vi "Eval X-Y-Z(a,t1,t2) Prep.vi"(0 "End":dbl[](array[numeric])=[1.0, 1.0] format="%.2f", 5 "Formulas":string[](array[string])=["", "", ""], 7 "Variables":string[](array[string])=["t1", "t2"], 9 "Parameters":cluster{string, dbl}[](array[cluster]) {"?" format="%.2f"}, 11 "Start":dbl[](array[numeric])=[0.0, 0.0] format="%.2f") -> (4 "Formulas":string[](array[string]), 6 "End":dbl[](array[numeric]) format="%.2f", 8 "time [msec]":u32, 10 "error (general)":bool, 12 "Variables":string[](array[string]), 13 "Start":dbl[](array[numeric]) format="%.2f", 14 "Parameters":cluster{string, dbl}[](array[cluster]) {"?" format="%.2f"}, 15 "specific error situation":bool)   [LabVIEW 2017, in "NI_Gmath.lvlib"]
uses:
  NI_Gmath.lvlib
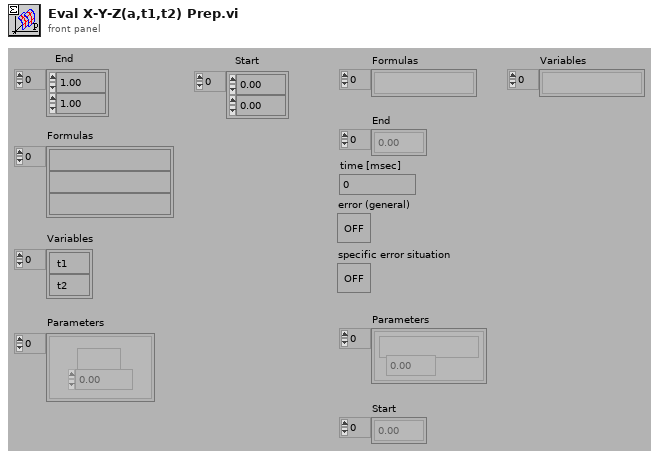
[diagram p1: front panel]
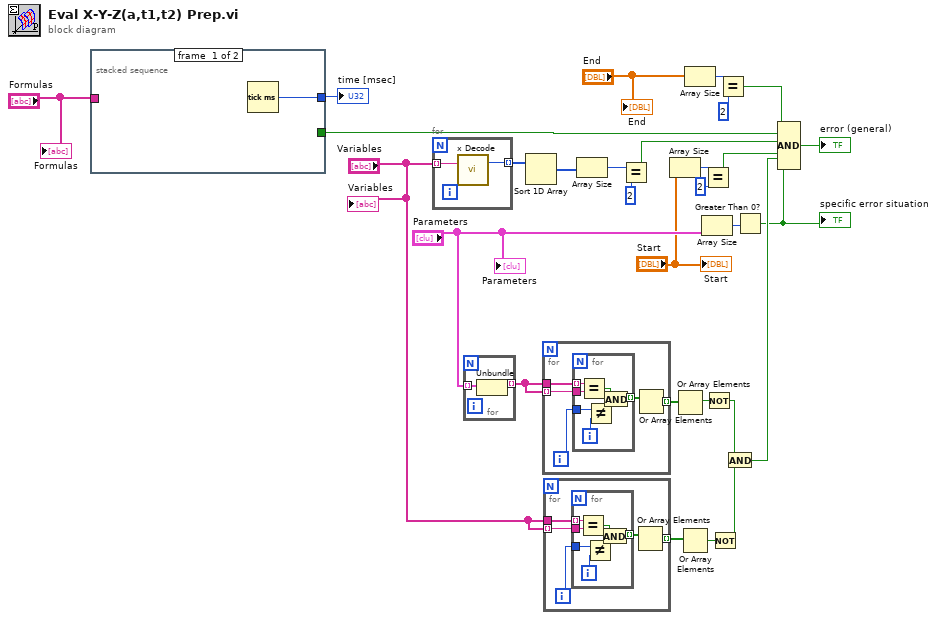
[diagram p0: block diagram]
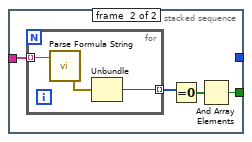
[diagram p2: hidden frame]
diagram:
  n1 = stacked-sequence {
    tunnel: [_ w31] -> w17
    tunnel: [w30 _] -> w11
    tunnel: "Formulas" -> [_ w33]
    frame #0 {
      n2 = Tick Count (ms)() -> (millisecond timer value=w30:u32)
    }
    frame #1 {
      n3 = for {
        tunnel: w33 -> [w37] mode=indexing
        tunnel: [w35] -> w32 mode=indexing
        n4 = call "Parse Formula String.vi"("formula"=w37) -> ("error out"=w36:errorcluster)  [unwired: 1 in, 1 out]
        n5 = Unbundle(w36) -> ("code"=w35:i32)  [unwired: 2 out]
      }
      n6 = Equal To 0?(x=w32) -> (x = 0?=w34:bool[])
      n7 = And Array Elements(Boolean array=w34) -> (logical AND=w31:bool)
    }
  }
  "time [msec]" <- w11
  n8 = for {
    tunnel: "Variables" -> [w39] mode=indexing
    tunnel: [w38] -> w1 mode=indexing
    n9 = call "x Decode.vi"("x string"=w39) -> ("number"=w38:i32)  [unwired: 1 in, 1 out]
  }
  n10 = for {
    tunnel: "Parameters" -> [w41] mode=indexing
    tunnel: [w40] -> w18 mode=indexing
    n11 = Unbundle(w41) -> (w40:string)  [unwired: 1 out]
  }
  n12 = Sort 1D Array(array=w1) -> (sorted array=w9:i32[])
  n13 = for {
    tunnel: w18 -> [w46]
    tunnel: w18 -> [w45] mode=indexing
    tunnel: [w42] -> w19 mode=indexing
    i -> [w44]
    n14 = for {
      tunnel: w46 -> [w53] mode=indexing
      tunnel: w45 -> [w52]
      tunnel: w44 -> [w51]
      tunnel: [w47] -> w43 mode=indexing
      i -> [w50]
      n15 = Equal?(x=w53, y=w52) -> (x = y?=w49:bool)
      n16 = Not Equal?(x=w51, y=w50) -> (x != y?=w48:bool)
      n17 = And(x=w49, y=w48) -> (x .and. y?=w47:bool)
    }
    n18 = Or Array Elements(Boolean array=w43) -> (logical OR=w42:bool)
  }
  n19 = for {
    tunnel: "Variables" -> [w58]
    tunnel: "Variables" -> [w57] mode=indexing
    tunnel: [w54] -> w24 mode=indexing
    i -> [w56]
    n20 = for {
      tunnel: w58 -> [w65] mode=indexing
      tunnel: w57 -> [w64]
      tunnel: w56 -> [w63]
      tunnel: [w59] -> w55 mode=indexing
      i -> [w62]
      n21 = Equal?(x=w65, y=w64) -> (x = y?=w61:bool)
      n22 = Not Equal?(x=w63, y=w62) -> (x != y?=w60:bool)
      n23 = And(x=w61, y=w60) -> (x .and. y?=w59:bool)
    }
    n24 = Or Array Elements(Boolean array=w55) -> (logical OR=w54:bool)
  }
  n25 = Array Size(array=w9) -> (size(s)=w8:i32)
  n26 = Equal?(x=w8, y=2) -> (x = y?=w16:bool)
  n27 = Array Size(array="Start") -> (size(s)=w5:i32)
  n28 = Or Array Elements(Boolean array=w19) -> (logical OR=w20:bool)
  n29 = Or Array Elements(Boolean array=w24) -> (logical OR=w25:bool)
  n30 = Array Size(array="End") -> (size(s)=w2:i32)
  n31 = Array Size(array="Parameters") -> (size(s)=w22:i32)
  n32 = Equal?(x=w5, y=2) -> (x = y?=w10:bool)
  n33 = Not(x=w20) -> (.not. x?=w27:bool)
  n34 = Not(x=w25) -> (.not. x?=w28:bool)
  n35 = Equal?(x=w2, y=2) -> (x = y?=w6:bool)
  n36 = And(x=w27, y=w28) -> (x .and. y?=w29:bool)
  n37 = Greater Than 0?(x=w22) -> (x > 0?=w23:bool)
  "specific error situation" <- w23
  n38 = Compound Arithmetic op=AND(w6, w17, w16, w10, w29, w23) -> (→"error (general)":bool)
  "Variables" <- "Variables"
  "Parameters" <- "Parameters"
  "Formulas" <- "Formulas"
  "Start" <- "Start"
  "End" <- "End"
